vi "Format Trace List.vi"(10 "Trace List Catalog":string) -> (2 "Trace List":string[][](array[string]))   [LabVIEW 2015]
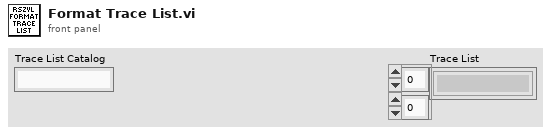
[diagram p1: front panel]
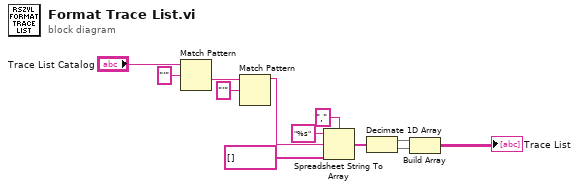
[diagram p0: block diagram]
diagram:
  n1 = Match Pattern(string="Trace List Catalog", regular expression="'") -> (after substring=w10:string)  [unwired: 1 in, 3 out]
  n2 = Match Pattern(string=w10, regular expression="'") -> (before substring=w9:string)  [unwired: 1 in, 3 out]
  n3 = Spreadsheet String To Array(delimiter (Tab)=",", format string="%s", spreadsheet string=w9, array type (2D Dbl)=string[] []) -> (array=w4:string[])
  n4 = Decimate 1D Array(w4) -> (w3:string[], w2:string[])
  n5 = Build Array(w3, w2) -> (→"Trace List":string[][])
